vi "6feladat.vi"() -> ()   [LabVIEW 2015]
panel:
  in  "U":dbl
  in  "f":dbl
  in  "A":dbl
  out "Waveform Chart 3":dbl[](graph)
  out "Waveform Chart 2":dbl[](graph)
  out "Waveform Chart":dbl[](graph)
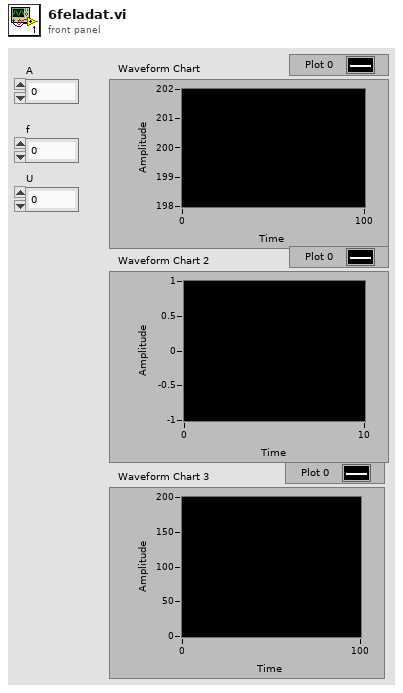
[diagram p1: front panel]
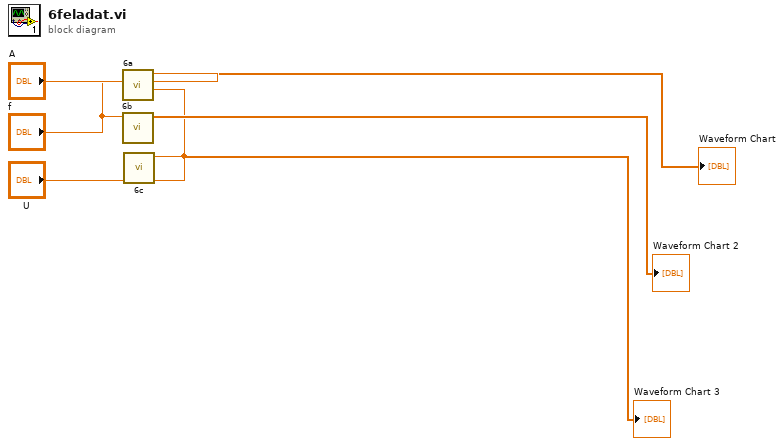
[diagram p0: block diagram]
diagram:
  n1 = call "6a.vi"("U"="U", "f"="f", "A"="A") -> ("Array"=→"Waveform Chart":dbl[])  [unwired: 8 in]
  n2 = call "6b.vi"("f"="f") -> ("Array"=→"Waveform Chart 2":dbl[])  [unwired: 10 in]
  n3 = call "6c.vi"("U"="U") -> ("Array"=→"Waveform Chart 3":dbl[])  [unwired: 10 in]
